vi "MicronGRPC Message.vi"(5 "Service Name":string, 6 "contextId":T1, 7 "Package Name":string, 8 "error in":errorcluster, 9 "timeout (ms)":i32=-1, 10 "Request Data":T4, 11 "gRPC ID":T1) -> (0 "error out":errorcluster, 2 "Response Data":T2, 3 "gRPC ID out":T1)   [LabVIEW 2019, in "MicronGRPCGeneratedClient.lvlib"]
uses:
  MicronGRPCGeneratedClient.lvlib
  <vilib>/gRPC/LabVIEW gRPC Library/Shared/grpcId.ctl
  RPC Messages/micronGrpc_MessageRequest.ctl
  RPC Messages/micronGrpc_MessageReply.ctl
  RPC Messages/micronGrpc_MessageReply_Status.ctl
  RPC Messages/micronGrpc_MessageReply_Flat.ctl
  RPC Messages/micronGrpc_MessageReply_Status_Flat.ctl
  14035477-4c25-4107-8ed5-d0c4ef420ce5.vi
  <vilib>/gRPC/LabVIEW gRPC Library/Shared/TranslateGrpcError.vi
  <vilib>/gRPC/LabVIEW gRPC Library/Shared/Wait On Occurrence.vi
  RPC Messages/FlatToRichmicronGrpc_MessageReply_Status.vi
  <vilib>/gRPC/LabVIEW gRPC Library/Shared/Is Feature Enabled.vi
  <vilib>/gRPC/LabVIEW gRPC Library/Server API/Server/Get Server DLL Path.vi
  <vilib>/Utility/error.llb/Error Cluster From Error Code.vi
  <vilib>/SLL Toolkit/SLL String/SLL String.lvlib
  <vilib>/gRPC/LabVIEW gRPC Library/grpc-lvsupport-release.lvlib
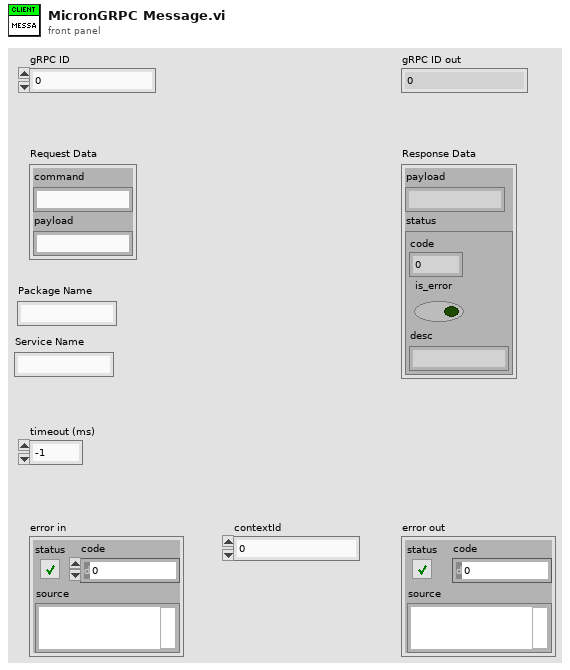
[diagram p1: front panel]
types:
  T1 = typedef "grpc-lvsupport-release.lvlib/grpcId.ctl" = u64
  T2 = typedef "MicronGRPCGeneratedClient.lvlib/micronGrpc_MessageReply.ctl" = cluster{"payload":string, "status":T3}
  T3 = typedef "MicronGRPCGeneratedClient.lvlib/micronGrpc_MessageReply_Status.ctl" = cluster{"code":i32, "is_error":bool, "desc":string}
  T4 = typedef "MicronGRPCGeneratedClient.lvlib/micronGrpc_MessageRequest.ctl" = cluster{"command":string, "payload":string}
  T5 = typedef "MicronGRPCGeneratedClient.lvlib/micronGrpc_MessageReply_Flat.ctl" = cluster{"payload":string, "status":T6}
  T6 = typedef "MicronGRPCGeneratedClient.lvlib/micronGrpc_MessageReply_Status_Flat.ctl" = cluster{"code":i32, "is_error":bool, "desc":string}
  T7 = typedef "MicronGRPCGeneratedClient.lvlib/micronGrpc_MessageRequest_Flat.ctl" = cluster{"command":string, "payload":string}
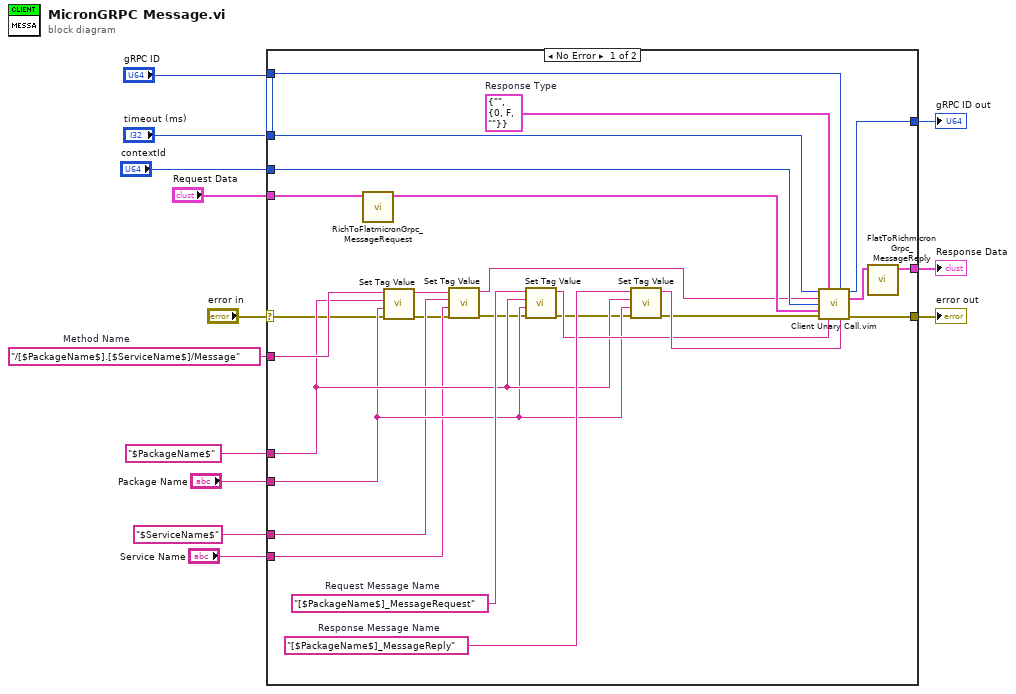
[diagram p0: block diagram]
diagram:
  w1 = "/[$PackageName$].[$ServiceName$]/Message"  # Method Name
  n1 = case shown="No Error" "error in" {
    selector: "error in" -> [w15 w40]
    tunnel: [w38 w40] -> w12
    tunnel: "gRPC ID" -> [w37 w41]
    tunnel: [w36 w41] -> w10
    tunnel: "Request Data" -> [w33 _]
    tunnel: [w30 _] -> w8
    tunnel: "timeout (ms)" -> [w35 _]
    tunnel: "contextId" -> [w34 _]
    tunnel: "$PackageName$" -> [w22 _]
    tunnel: "Package Name" -> [w21 _]
    tunnel: "$ServiceName$" -> [w20 _]
    tunnel: "Service Name" -> [w19 _]
    tunnel: w1 -> [w25 _]
    frame No Error {
      w29 = "[$PackageName$]_MessageReply"  # Response Message Name
      w27 = "[$PackageName$]_MessageRequest"  # Request Message Name
      w39 = T5 {"payload"="", "status"={"code"=0, "is_error"=FALSE, "desc"=""}}  # Response Type
      n2 = call "RichToFlatmicronGrpc_MessageRequest.vi"("InputCluster"=w33) -> ("OutputCluster"=w32:T7)  [unwired: 10 in]
      n3 = call <vilib>:"Set Tag Value.vi"("error in (no error)"=w15, "Tag Value"=w21, "Tag Name"=w22, "Input String"=w25) -> ("error out"=w18:errorcluster, "Output String"=w24:string)  [unwired: 6 in]
      n4 = call <vilib>:"Set Tag Value.vi"("error in (no error)"=w18, "Tag Value"=w19, "Tag Name"=w20, "Input String"=w24) -> ("error out"=w17:errorcluster, "Output String"=w23:string)  [unwired: 6 in]
      n5 = call <vilib>:"Set Tag Value.vi"("error in (no error)"=w17, "Tag Value"=w21, "Tag Name"=w22, "Input String"=w27) -> ("error out"=w16:errorcluster, "Output String"=w26:string)  [unwired: 6 in]
      n6 = call <vilib>:"Set Tag Value.vi"("error in (no error)"=w16, "Tag Value"=w21, "Tag Name"=w22, "Input String"=w29) -> ("error out"=w14:errorcluster, "Output String"=w28:string)  [unwired: 6 in]
      n7 = call "Client Unary Call.vim"("ClientID in"=w37, "Response Type"=w39, "timeout (ms)"=w35, "Method Name"=w23, "contextId"=w34, "Request Data"=w32, "error in"=w14, "Request Message Name"=w26, "Response Message Name"=w28) -> ("ClientID out"=w36:u64, "Response Data"=w31:T5, "error out"=w38:errorcluster)  [unwired: 4 in]
      n8 = call "FlatToRichmicronGrpc_MessageReply.vi"("InputCluster"=w31) -> ("OutputCluster"=w30:T2)  [unwired: 10 in]
    }
    frame Error {
    }
  }
  "error out" <- w12
  "gRPC ID out" <- w10
  "Response Data" <- w8
